vi "add.vi"(9 "y":dbl, 11 "x":dbl) -> (2 "x+y":dbl)   [LabVIEW 2012]
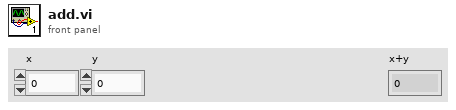
[diagram p1: front panel]
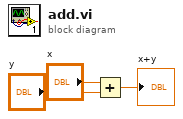
[diagram p0: block diagram]
diagram:
  n1 = Add(x="x", y="y") -> (x+y=→"x+y":dbl)
